vi "Error Query.vi"(8 "error in (no error)":errorcluster, 11 "VISA resource name":refnum<visa-resource-name>) -> (0 "error out":errorcluster, 1 "Error Message":string, 3 "VISA resource name out":refnum<visa-resource-name>)   [LabVIEW 2025, in "NewtonsPSM1735.lvlib"]
doc: "Queries the instrument for any errors in the instrument's error queue. It will continue to read errors until all errors have been read from the instrument. Any errors will be returned in the <B>error out</B> control.\n\n<B>Note:</B>\nThis VI is called automatically by most driver VIs so it is not usually necessary to call this in an application."
uses:
  NewtonsPSM1735.lvlib
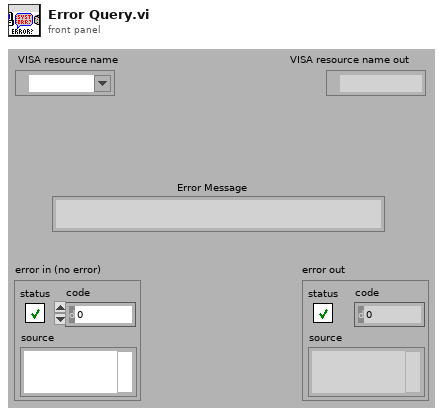
[diagram p1: front panel]
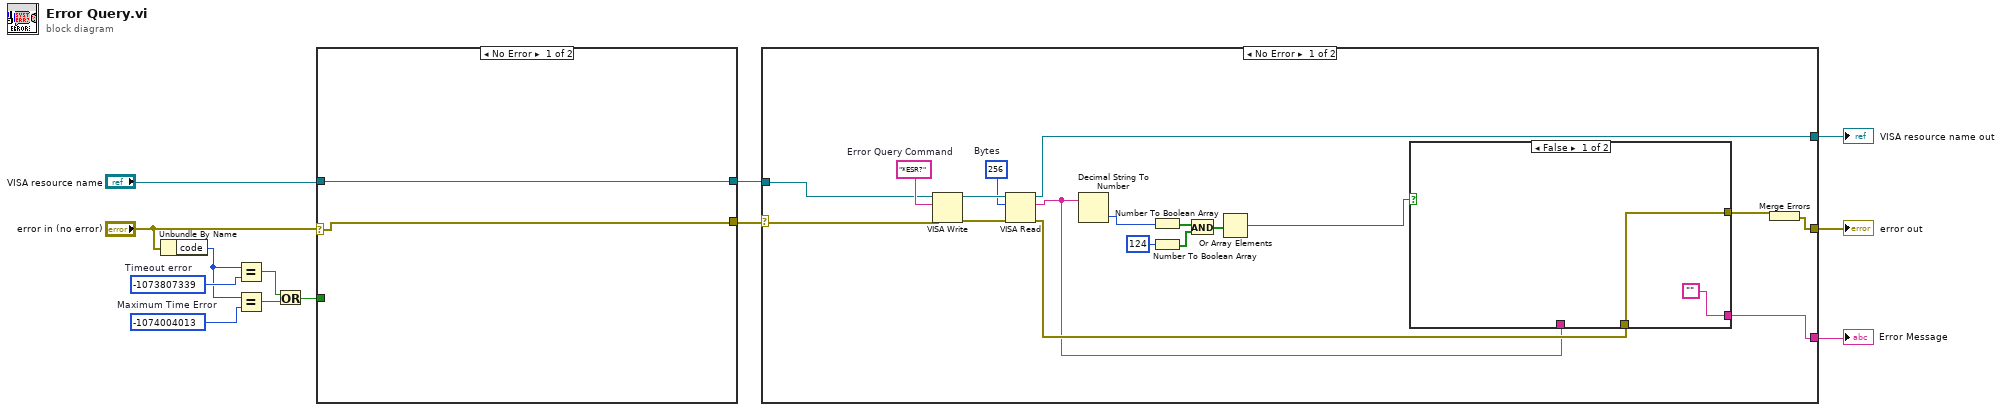
[diagram p0: block diagram]
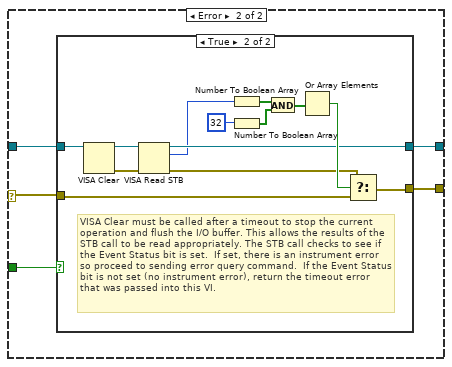
[diagram p2: hidden frame]
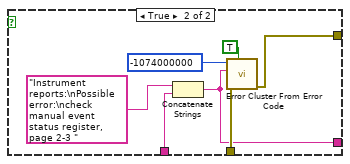
[diagram p4: hidden frame]
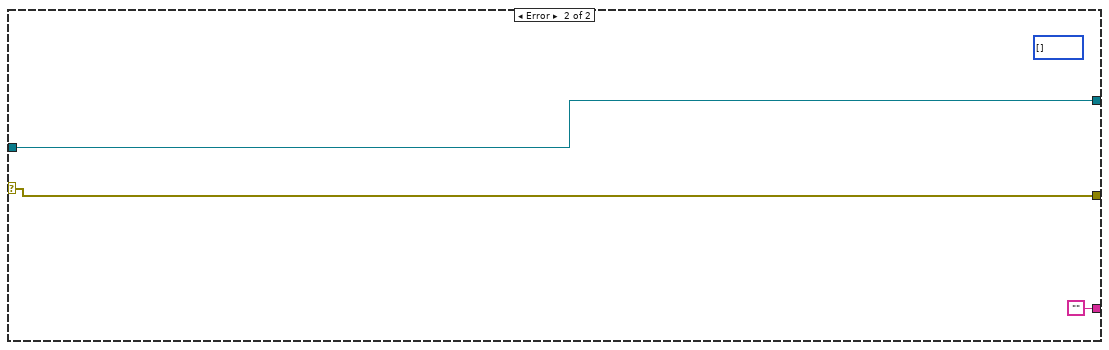
[diagram p5: hidden frame]
diagram:
  w5 = -1074004013  # Maximum Time Error
  w7 = -1073807339  # Timeout error
  n1 = Unbundle By Name("error in (no error)") -> ("code"=w6:i32)
  n2 = Equal?(x=w6, y=w7) -> (x = y?=w3:bool)
  n3 = Equal?(x=w6, y=w5) -> (x = y?=w4:bool)
  n4 = Or(x=w3, y=w4) -> (x .or. y?=w2:bool)
  n5 = case shown="No Error" "error in (no error)" {
    selector: "error in (no error)" -> [w14 w18]
    tunnel: "VISA resource name" -> [w15 w20]
    tunnel: [w15 w19] -> w9
    tunnel: [w14 w17] -> w10
    tunnel: w2 -> [_ w16]
    frame No Error {
    }
    frame Error {
      n6 = case shown="True" w16 {
        tunnel: w20 -> [w22 w28]
        tunnel: [w22 w25] -> w19
        tunnel: w18 -> [w21 w31]
        tunnel: [w21 w30] -> w17
        frame False {
          # "Error code not a timeout, so best to pass on to user."
        }
        frame True {
          # "VISA Clear must be called after a timeout to stop the current operation and flush the I/O buffer. This allows the results of the  STB call to be read appropriately. The STB call checks to see if the Event Status bit is set.  If set, there is an instrument error so proceed to sending error query command.  If the Event Status bit is not set (no instrument error), return the timeout error that was passed into this VI."
          n7 = VISA Clear(VISA resource name=w28) -> (VISA resource name out=w27:refnum<visa-resource-name>, error out=w26:errorcluster)  [unwired: 1 in]
          n8 = VISA Read STB(8:w26, 11:w27) -> (0:w24:errorcluster, 2:w23:u16, 3:w25:refnum<visa-resource-name>)
          n9 = Number To Boolean Array(number=w23) -> (Boolean array=w32:bool[])
          n10 = Number To Boolean Array(number=32) -> (Boolean array=w34:bool[])
          n11 = And(x=w32, y=w34) -> (x .and. y?=w33:bool[])
          n12 = Or Array Elements(Boolean array=w33) -> (logical OR=w29:bool)
          n13 = Select(t=w24, s=w29, f=w31) -> (s? t:f=w30:errorcluster)
        }
      }
    }
  }
  n14 = case shown="No Error" w10 {
    selector: w10 -> [w37 w63]
    tunnel: [w41 w65] -> w13
    tunnel: w9 -> [w36 w65]
    tunnel: [w53 w63] -> w12
    tunnel: [w40 ""] -> w11
    frame No Error {
      w50 = u32 256  # Bytes
      w48 = "*ESR?"  # Error Query Command
      n15 = VISA Write(VISA resource name=w36, write buffer=w48, error in (no error)=w37) -> (VISA resource name out=w51:refnum<visa-resource-name>, error out=w49:errorcluster)  [unwired: 1 out]
      n16 = VISA Read(VISA resource name=w51, byte count=w50, error in (no error)=w49) -> (VISA resource name out=w41:refnum<visa-resource-name>, read buffer=w38:string, error out=w42:errorcluster)  [unwired: 1 out]
      n17 = Decimal String To Number(string=w38) -> (number=w39:i32)  [unwired: 3 out]
      n18 = Number To Boolean Array(number=w39) -> (Boolean array=w44:bool[])
      n19 = Number To Boolean Array(number=124) -> (Boolean array=w46:bool[])
      n20 = And(x=w44, y=w46) -> (x .and. y?=w45:bool[])
      n21 = Or Array Elements(Boolean array=w45) -> (logical OR=w43:bool)
      n22 = case shown="False" w43 {
        tunnel: [w55 w56] -> w52
        tunnel: w42 -> [w55 w60]
        tunnel: ["" w59] -> w40
        tunnel: w38 -> [_ w57]
        frame False {
        }
        frame True {
          n23 = Concatenate Strings("Instrument reports:\nPossible error:\ncheck manual event status register, page 2-3 " ("Source"), w57) -> (w59:string)
          n24 = call <vilib>:"Error Cluster From Error Code.vi"("show call chain? (False)"=TRUE, "error in (no error)"=w60, "error message (\"\")"=w59, "error code (0)"=-1074000000 ("Code")) -> ("error out"=w56:errorcluster)  [unwired: 5 out]
        }
      }
      n25 = Merge Errors(w52) -> (w53:errorcluster)
    }
    frame Error {
      (unwired) i32[] []
    }
  }
  "VISA resource name out" <- w13
  "error out" <- w12
  "Error Message" <- w11
